vi "Set_DO.vi"(0 "reference in":refnum<class "Sig_DO_Simple.lvclass">, 5 "DO":bool, 11 "error in (no error)":errorcluster) -> (4 "reference out":refnum<class "Sig_DO_Simple.lvclass">, 15 "error out":errorcluster)   [LabVIEW 2019, in "Sig_DO_Simple.lvclass"]
uses:
  Sig_DO_Simple.lvclass
  D:/H4000/src/Proccess_class/Proccess.lvclass
  Sig_DO_Simple.lvclass/Sig_DO_Simple.ctl
  Proccess_class/Proccess.lvclass/Proccess.ctl
  Proccess_class/Read TagName.vi
  Proccess_class/Read Logger.vi
  Logger_class/WriteEvent.vi
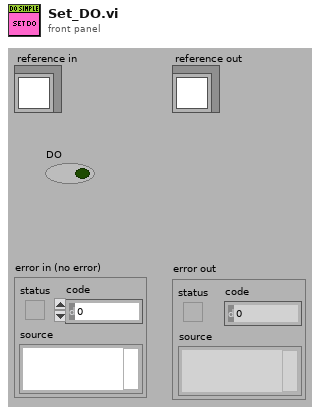
[diagram p1: front panel]
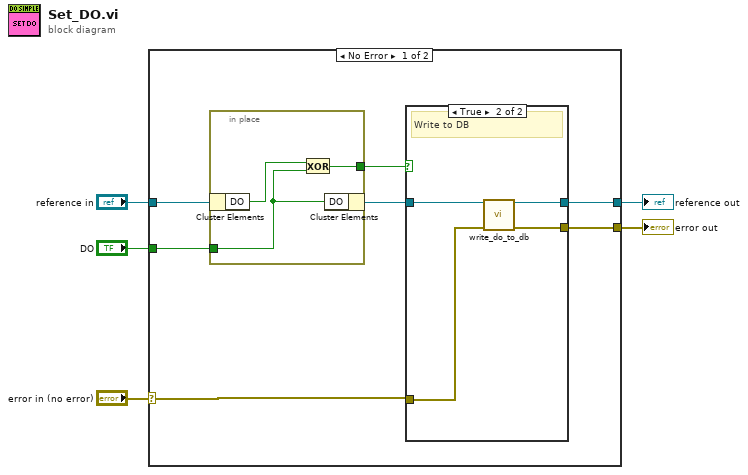
[diagram p0: block diagram]
diagram:
  n1 = case shown="No Error" "error in (no error)" {
    selector: "error in (no error)" -> [w12 w23]
    tunnel: [w10 w23] -> w4
    tunnel: [w11 w22] -> w2
    tunnel: "reference in" -> [w7 w22]
    tunnel: "DO" -> [w8 _]
    frame No Error {
      n2 = in-place {
        in-place-border: w8 -> [w21]
        in-place-border: [w20] -> w9
        n3 = in-place-cluster #1(w7) -> ("DO"=w19:bool)
        n4 = Exclusive Or(1:w21, 2:w19) -> (0:w20:bool)
        n5 = in-place-cluster #1("DO"=w21) -> (w6:refnum<class "Sig_DO_Simple.lvclass">)
      }
      n6 = case shown="True" w9 {
        tunnel: w6 -> [w14 w16]
        tunnel: [w14 w18] -> w11
        tunnel: w12 -> [w13 w15]
        tunnel: [w13 w17] -> w10
        frame False {
        }
        frame True {
          # "Write to DB"
          n7 = call "write_do_to_db.vi"("reference in"=w16, "error in (no error)"=w15) -> ("reference out"=w18:refnum<class "Sig_DO_Simple.lvclass">, "error out"=w17:errorcluster)  [unwired: 12 in]
        }
      }
    }
    frame Error {
    }
  }
  "error out" <- w4
  "reference out" <- w2
